vi "Read_Xbox-Controller.vi"() -> ()   [LabVIEW 2018]
uses:
  <vilib>/Utility/inputDevices.llb/joystickAcquire.vi
  <vilib>/Utility/inputDevices.llb/closeJoystick.vi
panel:
  out "appended array":dbl[](array[numeric])
  out "RightOutput-":dbl
  out "RightOutput+":dbl
  out "LeftOutput-":dbl
  out "LeftOutput+":dbl
  out "RightStick":dbl
  out "LeftStick":dbl
  in  "RightStick Deadzone +":dbl=2000.0
  in  "RightStick Deadzone -":dbl=-250.0
  in  "LeftStick Deadzone +":dbl=2700.0
  in  "LeftStick Deadzone -":dbl
  out "array":i32[](array[numeric])=[289, 1907, -32768, 34, 2313, -32768, 0, 0]
  in  "stop":bool
  out "error out":errorcluster
  out "direction info":T1={"pov 1"=-1, "pov 2"=-1, "pov 3"=-1, "pov 4"=-1}
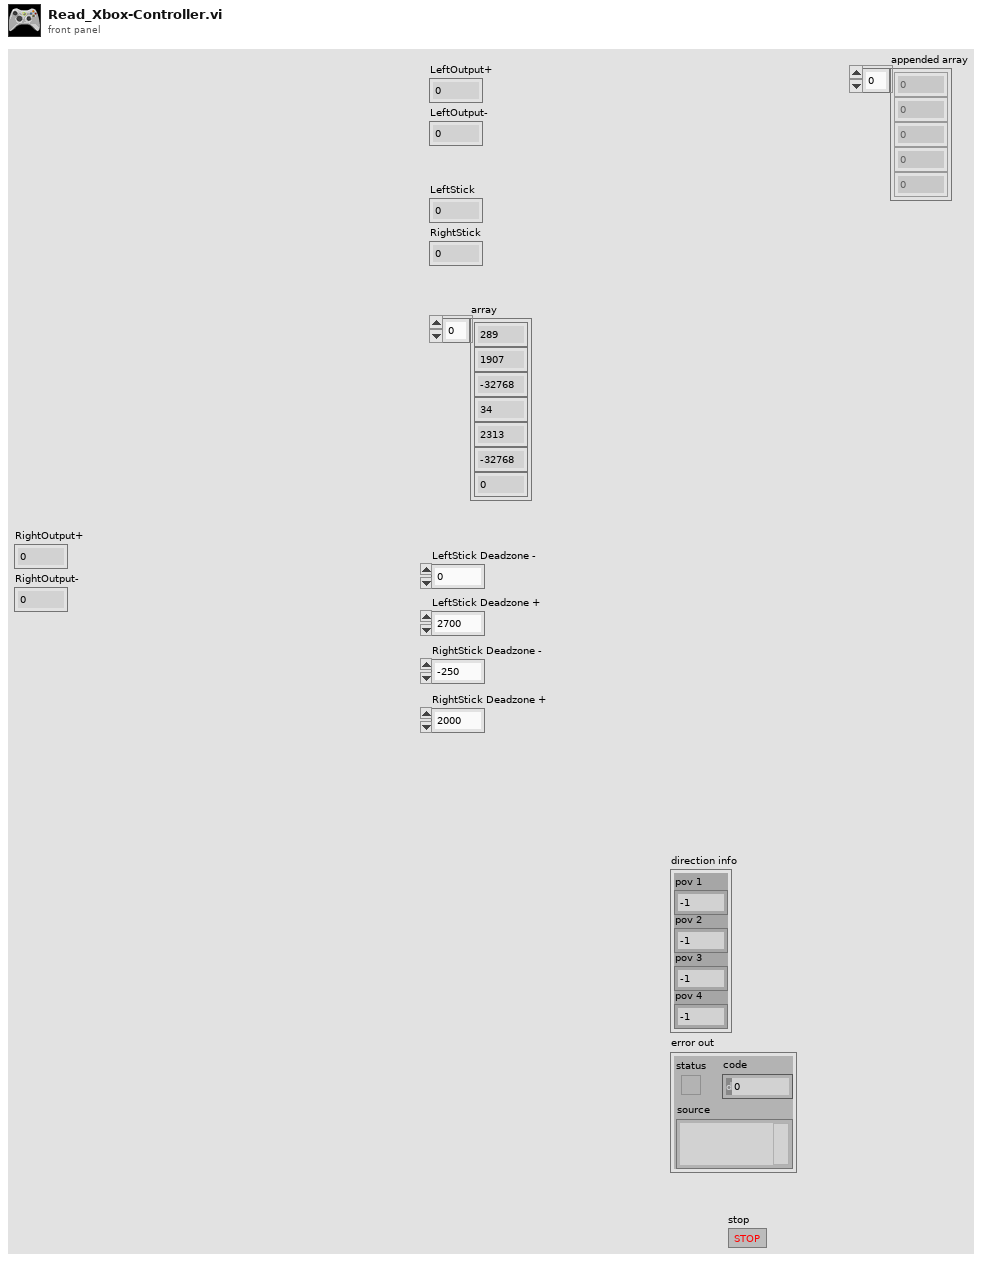
[diagram p1: front panel]
types:
  T1 = cluster{"pov 1":i32, "pov 2":i32, "pov 3":i32, "pov 4":i32}
  T2 = cluster{"X axis":i32, "Y axis":i32, "Z axis":i32, "X axis rotation":i32, "Y axis rotation":i32, "Z axis rotation":i32, "U axis":i32, "V axis":i32}
  T3 = cluster{"button 1":bool, "button 2":bool, "button 3":bool, "button 4":bool, "button 5":bool, "button 6":bool, "button 7":bool, "button 8":bool, "button 9":bool, "button 10":bool, "button 11":bool, "button 12":bool, "button 13":bool, "button 14":bool, "button 15":bool, "button 16":bool, "button 17":bool, "button 18":bool, "button 19":bool, "button 20":bool, "button 21":bool, "button 22":bool, "button 23":bool, "button 24":bool, "button 25":bool, "button 26":bool, "button 27":bool, "button 28":bool, "button 29":bool, "button 30":bool, "button 31":bool, "button 32":bool}
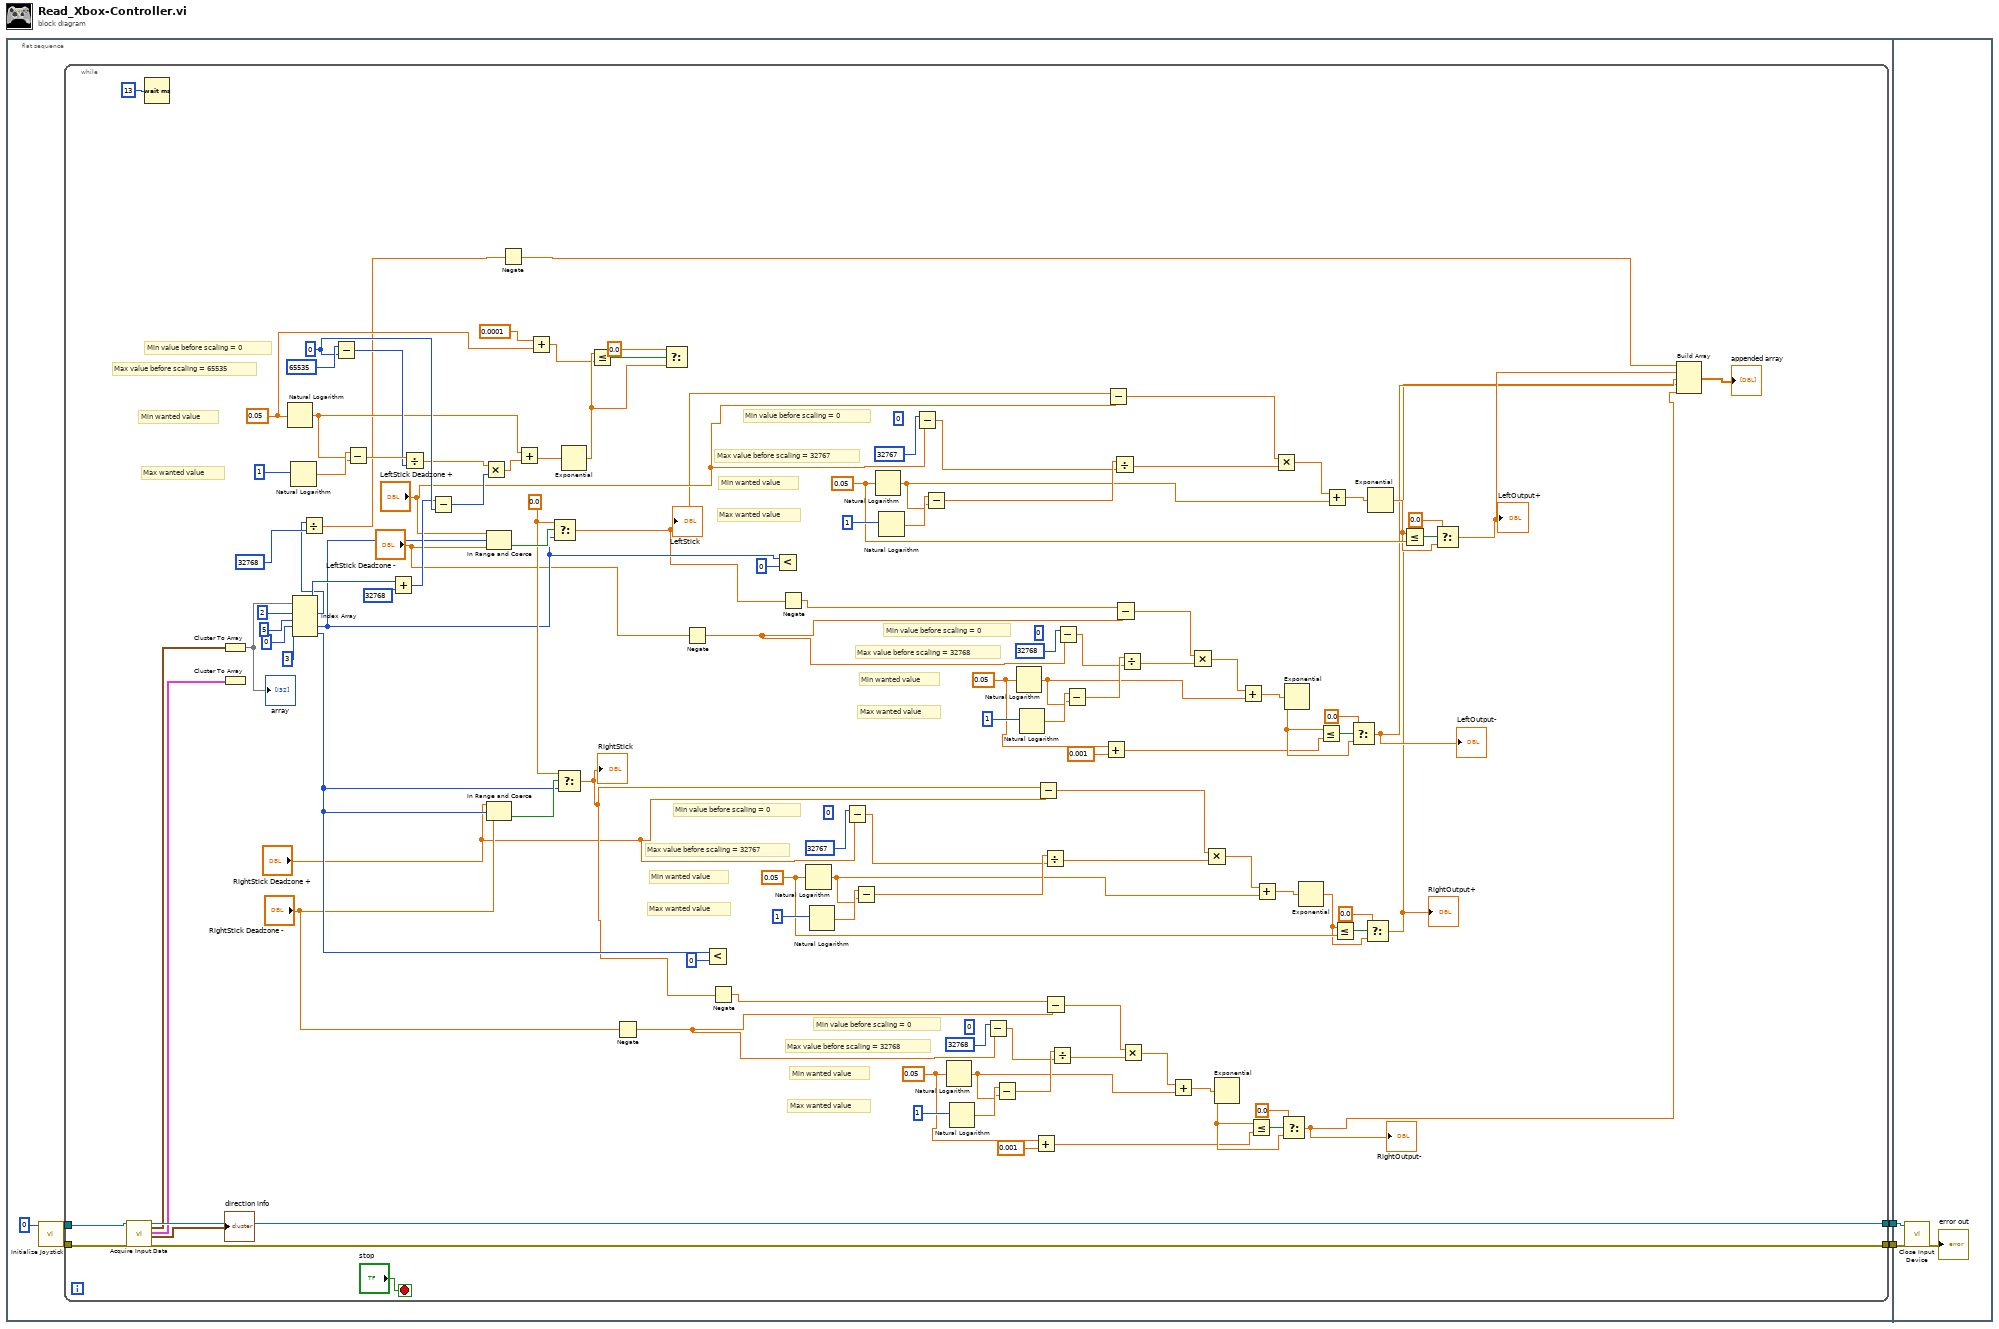
[diagram p0: block diagram]
diagram:
  n1 = flat-sequence {
    tunnel: [w5] -> w2
    tunnel: [w4] -> w1
    tunnel: w2 -> [w130]
    tunnel: w1 -> [w129]
    frame #0 {
      n2 = call <vilib>:"Initialize Joystick.vi"("device index"=0) -> ("error out"=w6:errorcluster, "device ID"=w7:refnum<k1>)  [unwired: 9 in]
      n3 = while {
        tunnel: w7 -> [w126]
        tunnel: w6 -> [w125]
        tunnel: [w124] -> w5
        tunnel: [w122] -> w4
        stop <- "stop" stop-if-true
        w23 = 0.05 ("x")
        (unwired) 0 ("index")
        w43 = 0.05 ("x")
        (unwired) 0 ("index")
        w56 = 0.05 ("x")
        (unwired) 0 ("index")
        w79 = 0.05 ("x")
        (unwired) 0 ("index")
        w91 = 0.0 ("t")
        w98 = 0.05 ("x")
        w112 = 0 ("index")
        # "Min wanted value"
        # "Max wanted value"
        # "Max value before scaling = 32768"
        # "Min value before scaling = 0"
        # "Min wanted value"
        # "Max wanted value"
        # "Max value before scaling = 32767"
        # "Min value before scaling = 0"
        # "Min wanted value"
        # "Max wanted value"
        # "Max value before scaling = 32768"
        # "Min value before scaling = 0"
        # "Min wanted value"
        # "Max wanted value"
        # "Max value before scaling = 32767"
        # "Min value before scaling = 0"
        # "Min wanted value"
        # "Max wanted value"
        # "Max value before scaling = 65535"
        # "Min value before scaling = 0"
        n4 = call-poly <vilib>:"Acquire Input Data.vi"("device ID"=w126, "error in (no error)"=w125) -> ("device ID"=w124:refnum<k1>, "axis info"=w121:T2, "button info"=w120:T3, "direction info"=→"direction info":T1, "error out"=w122:errorcluster)  [unwired: 13 in]
        n5 = Wait (ms)(milliseconds to wait=u32 13) -> ()  [unwired: 1 out]
        n6 = Cluster To Array(cluster=w121) -> (array=w119:i32[])
        "array" <- w119
        n7 = Cluster To Array(cluster=w120) -> ()  [unwired: 1 out]
        n8 = Natural Logarithm(1:w98) -> (0:w108:dbl)
        n9 = Natural Logarithm(1:1 ("index")) -> (0:w116:dbl)
        n10 = Index Array(array=w119, index #1=2 ("index"), index #2=5 ("index"), index #3=0 ("index"), index #4=3 ("index")) -> (element #1=w10:i32, element #2=w104:i32, element #3=w61:i32, element #4=w20:i32)
        n11 = Divide(x=w10, y=32768) -> (x/y=w9:dbl)
        n12 = Subtract(x=65535 ("index"), y=w112) -> (x-y=w113:i32)
        n13 = Subtract(x=w116, y=w108) -> (x-y=w115:dbl)
        n14 = Add(x=w104, y=32768) -> (x+y=w103:i32)
        n15 = Divide(x=w115, y=w113) -> (x/y=w110:dbl)
        n16 = Subtract(x=w103, y=w112) -> (x-y=w111:i32)
        n17 = Multiply(x=w110, y=w111) -> (x*y=w109:dbl)
        n18 = In Range and Coerce(upper limit="LeftStick Deadzone +", x=w61, lower limit="LeftStick Deadzone -") -> (In Range?=w92:bool)  [unwired: 1 out]
        n19 = In Range and Coerce(upper limit="RightStick Deadzone +", x=w20, lower limit="RightStick Deadzone -") -> (In Range?=w93:bool)  [unwired: 1 out]
        n20 = Negate(x=w9) -> (-x=w8:dbl)
        n21 = Add(x=w108, y=w109) -> (x+y=w107:dbl)
        n22 = Add(x=0.0001 ("y"), y=w98) -> (x+y=w96:dbl)
        n23 = Select(t=w91, s=w92, f=w61) -> (s? t:f=w60:dbl)
        "LeftStick" <- w60
        n24 = Select(t=w91, s=w93, f=w20) -> (s? t:f=w19:dbl)
        "RightStick" <- w19
        n25 = Exponential(1:w107) -> (0:w99:dbl)
        n26 = Less Or Equal?(x=w99, y=w96) -> (x <= y?=w101:bool)
        n27 = Negate(x="RightStick Deadzone -") -> (-x=w24:dbl)
        n28 = Select(t=0.0, s=w101, f=w99) -> ()  [unwired: 1 out]
        n29 = Negate(x="LeftStick Deadzone -") -> (-x=w57:dbl)
        n30 = Less?(x=w20, y=0) -> ()  [unwired: 1 out]
        n31 = Negate(x=w19) -> (-x=w25:dbl)
        n32 = Less?(x=w61, y=0) -> ()  [unwired: 1 out]
        n33 = Negate(x=w60) -> (-x=w59:dbl)
        n34 = Natural Logarithm(1:w43) -> (0:w45:dbl)
        n35 = Natural Logarithm(1:1 ("index")) -> (0:w51:dbl)
        n36 = Subtract(x=32767 ("index"), y="RightStick Deadzone +") -> (x-y=w49:dbl)
        n37 = Subtract(x=w51, y=w45) -> (x-y=w50:dbl)
        n38 = Natural Logarithm(1:w79) -> (0:w81:dbl)
        n39 = Natural Logarithm(1:1 ("index")) -> (0:w88:dbl)
        n40 = Subtract(x=32767 ("index"), y="LeftStick Deadzone +") -> (x-y=w86:dbl)
        n41 = Subtract(x=w88, y=w81) -> (x-y=w87:dbl)
        n42 = Natural Logarithm(1:w23) -> (0:w30:dbl)
        n43 = Natural Logarithm(1:1 ("index")) -> (0:w36:dbl)
        n44 = Subtract(x=32768 ("index"), y=w24) -> (x-y=w34:dbl)
        n45 = Subtract(x=w36, y=w30) -> (x-y=w35:dbl)
        n46 = Natural Logarithm(1:w56) -> (0:w66:dbl)
        n47 = Natural Logarithm(1:1 ("index")) -> (0:w72:dbl)
        n48 = Add(x=w23, y=0.001) -> (x+y=w21:dbl)
        n49 = Subtract(x=w19, y="RightStick Deadzone +") -> (x-y=w48:dbl)
        n50 = Divide(x=w50, y=w49) -> (x/y=w47:dbl)
        n51 = Subtract(x=w25, y=w24) -> (x-y=w33:dbl)
        n52 = Divide(x=w35, y=w34) -> (x/y=w32:dbl)
        n53 = Subtract(x=32768 ("index"), y=w57) -> (x-y=w70:dbl)
        n54 = Subtract(x=w72, y=w66) -> (x-y=w71:dbl)
        n55 = Add(x=w56, y=0.001) -> (x+y=w54:dbl)
        n56 = Subtract(x=w60, y="LeftStick Deadzone +") -> (x-y=w84:dbl)
        n57 = Divide(x=w87, y=w86) -> (x/y=w83:dbl)
        n58 = Subtract(x=w59, y=w57) -> (x-y=w69:dbl)
        n59 = Divide(x=w71, y=w70) -> (x/y=w68:dbl)
        n60 = Multiply(x=w33, y=w32) -> (x*y=w31:dbl)
        n61 = Add(x=w31, y=w30) -> (x+y=w29:dbl)
        n62 = Multiply(x=w69, y=w68) -> (x*y=w67:dbl)
        n63 = Multiply(x=w48, y=w47) -> (x*y=w46:dbl)
        n64 = Exponential(1:w29) -> (0:w26:dbl)
        n65 = Add(x=w67, y=w66) -> (x+y=w65:dbl)
        n66 = Less Or Equal?(x=w26, y=w21) -> (x <= y?=w28:bool)
        n67 = Add(x=w46, y=w45) -> (x+y=w44:dbl)
        n68 = Multiply(x=w84, y=w83) -> (x*y=w82:dbl)
        n69 = Select(t=0.0, s=w28, f=w26) -> (s? t:f=w12:dbl)
        "RightOutput-" <- w12
        n70 = Exponential(1:w65) -> (0:w62:dbl)
        n71 = Exponential(1:w44) -> (0:w40:dbl)
        n72 = Less Or Equal?(x=w62, y=w54) -> (x <= y?=w64:bool)
        n73 = Add(x=w82, y=w81) -> (x+y=w80:dbl)
        n74 = Less Or Equal?(x=w40, y=w43) -> (x <= y?=w42:bool)
        n75 = Select(t=0.0, s=w64, f=w62) -> (s? t:f=w14:dbl)
        "LeftOutput-" <- w14
        n76 = Select(t=0.0, s=w42, f=w40) -> (s? t:f=w13:dbl)
        "RightOutput+" <- w13
        n77 = Exponential(1:w80) -> (0:w76:dbl)
        n78 = Less Or Equal?(x=w76, y=w79) -> (x <= y?=w78:bool)
        n79 = Select(t=0.0, s=w78, f=w76) -> (s? t:f=w15:dbl)
        "LeftOutput+" <- w15
        n80 = Build Array(w8, w15, w14, w13, w12) -> (→"appended array":dbl[])
      }
    }
    frame #1 {
      n81 = call-poly <vilib>:"Close Input Device.vi"("error in (no error)"=w129, "device ID"=w130) -> ("error out"=→"error out":errorcluster)  [unwired: 8 in]
    }
  }
